vi "clear status flag.vi"(8 "error in (no error)":errorcluster, 10 "flag name to clear":string, 11 "flag to clear":u32 format="%x") -> (0 "error out":errorcluster)   [LabVIEW 2024, in "atsj peakcan basic.lvlib"]
uses:
  atsj peakcan basic.lvlib
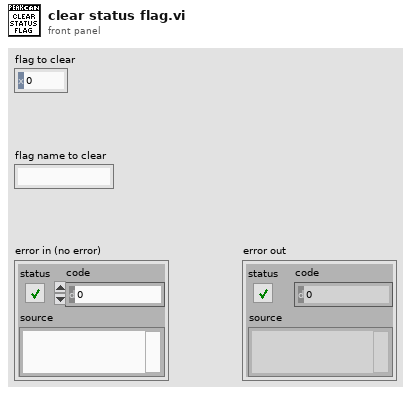
[diagram p1: front panel]
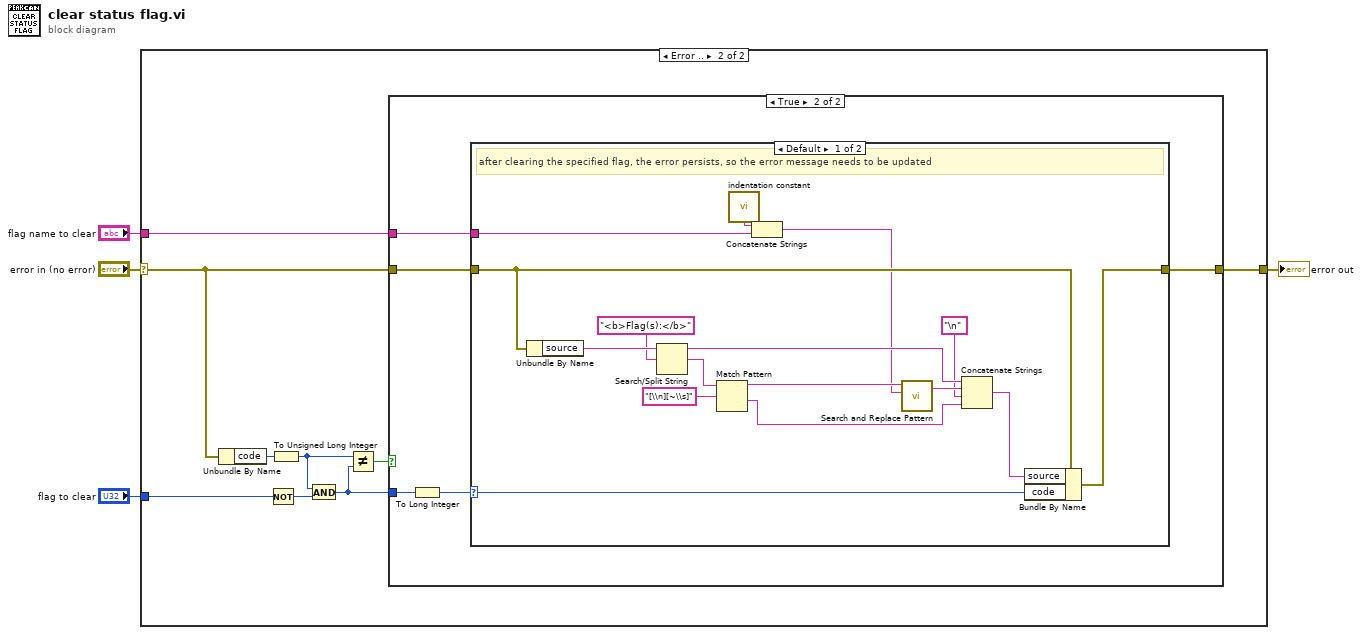
[diagram p0: block diagram]
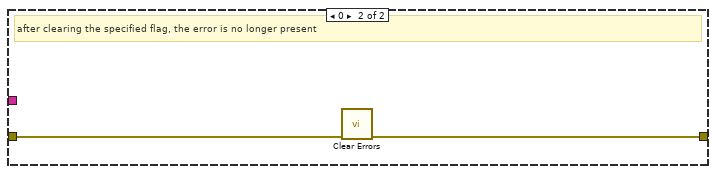
[diagram p4: hidden frame]
diagram:
  n1 = case shown="Error .." "error in (no error)" {
    selector: "error in (no error)" -> [w5 w7]
    tunnel: "flag to clear" -> [_ w13]
    tunnel: "flag name to clear" -> [_ w8]
    tunnel: [w5 w6] -> w1
    frame No Error {
    }
    frame Error {
      n2 = Unbundle By Name(w7) -> ("code"=w10:i32)
      n3 = Not(x=w13) -> (.not. x?=w14:u32)
      n4 = To Unsigned Long Integer(number=w10) -> (unsigned 32bit integer=w12:u32)
      n5 = And(x=w12, y=w14) -> (x .and. y?=w9:u32)
      n6 = Not Equal?(x=w12, y=w9) -> (x != y?=w11:bool)
      n7 = case shown="True" w11 {
        tunnel: w7 -> [w15 w18]
        tunnel: w9 -> [_ w20]
        tunnel: [w15 w17] -> w6
        tunnel: w8 -> [_ w16]
        frame False {
        }
        frame True {
          n8 = To Long Integer(number=w20) -> (32bit integer=w19:i32)
          n9 = case shown="Default" w19 {
            selector: w19 -> [w27 _]
            tunnel: w18 -> [w29 w38]
            tunnel: [w28 w37] -> w17
            tunnel: w16 -> [w31 _]
            frame Default {
              # "after clearing the specified flag, the error persists, so the error message needs to be updated"
              n10 = Unbundle By Name(w29) -> ("source"=w36:string)
              n11 = Search/Split String(string=w36, search string/char (-)="<b>Flag(s):</b>") -> (substring before match=w24:string, match + rest of string=w34:string)  [unwired: 1 in, 1 out]
              n12 = Match Pattern(string=w34, regular expression="[\\n][~\\s]") -> (before substring=w35:string, after substring=w25:string)  [unwired: 1 in, 2 out]
              n13 = call "indentation constant.vi"() -> ("indentation"=w30:string)
              n14 = Concatenate Strings(w30, w31) -> (w21:string)
              n15 = call <vilib>:"Search and Replace Pattern.vi"("string"=w35, "regular expression (\"\")"=w21) -> ("result string"=w26:string)  [unwired: 3 in, 1 out]
              n16 = Concatenate Strings(w24, w26, "\n", w25) -> (w23:string)
              n17 = Bundle By Name(cluster=w29, "source"=w23, "code"=w27) -> (w28:errorcluster)
            }
            frame 0 {
              # "after clearing the specified flag, the error is no longer present"
              n18 = call <vilib>:"Clear Errors.vi"("error in (no error)"=w38) -> ("error out"=w37:errorcluster)  [unwired: 5 in, 1 out]
            }
          }
        }
      }
    }
  }
  "error out" <- w1
